vi "setTelemetry.vi"(10 "Telemetry":refnum<class "Telemetry.lvclass">, 11 "Model in":refnum<class "Model.lvclass">) -> (3 "Model out":refnum<class "Model.lvclass">)   [LabVIEW 2016, in "Model.lvclass"]
uses:
  Model.lvclass
  Telemetry/Telemetry.lvclass
  Model.lvclass/Model.ctl
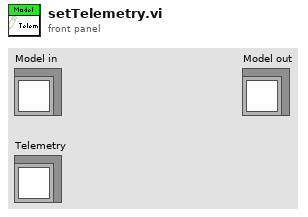
[diagram p1: front panel]
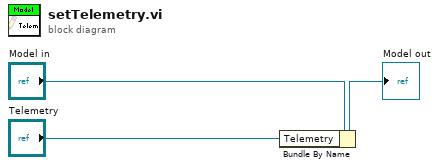
[diagram p0: block diagram]
diagram:
  n1 = Bundle By Name(cluster="Model in", "Telemetry"="Telemetry") -> (→"Model out":refnum<class "Model.lvclass">)
